vi "_시리얼 데이타 전송.vi"(2 "전송 문자열":string="FPGARX 0 1", 3 "시리얼 포트":refnum<visa-resource-name>) -> (0 "Processing Time(ms)":u32, 1 "송신 실패(T)":bool)   [LabVIEW 2015]
panel:
  out "에러 출력":errorcluster
  out "수신 문자열 버퍼":string
  out "수신 타이머 값":u32
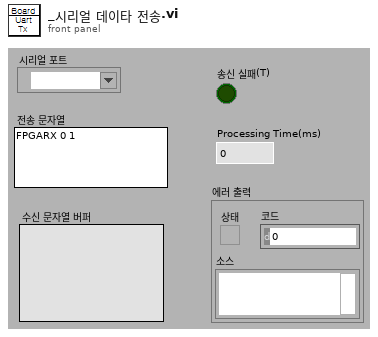
[diagram p1: front panel]
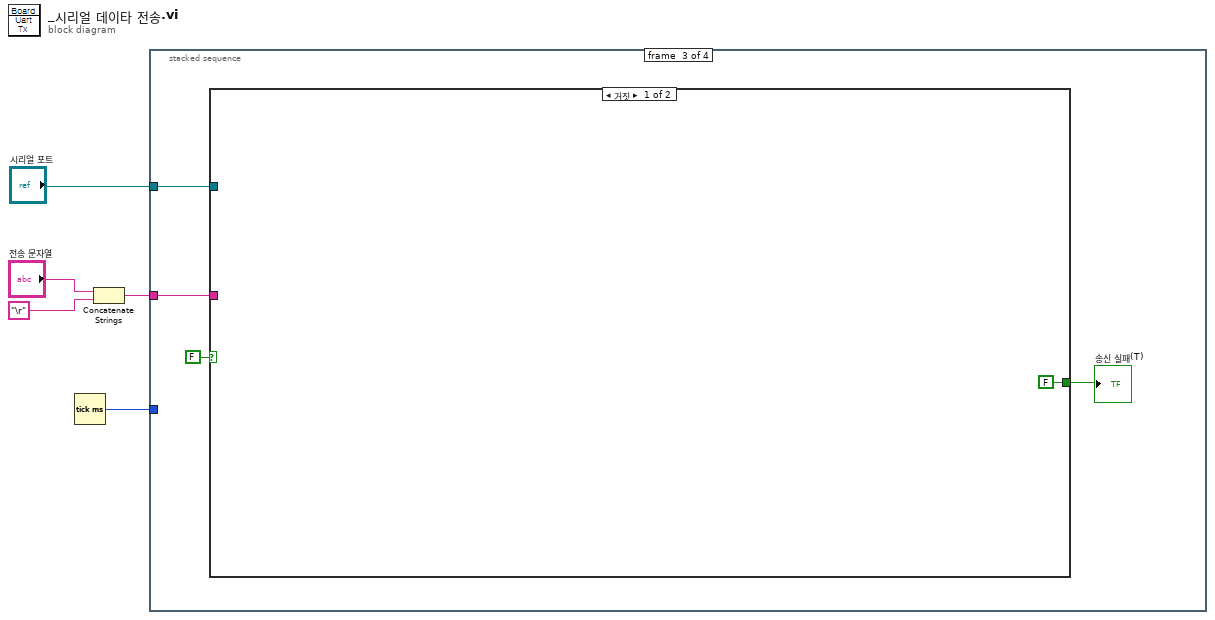
[diagram p0: block diagram]
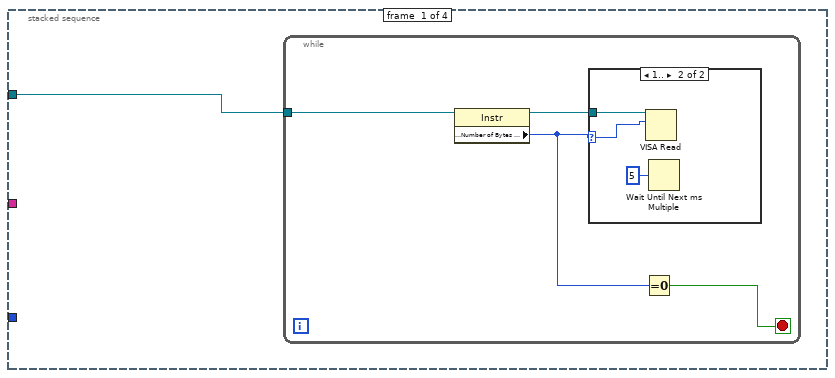
[diagram p2: hidden frame]
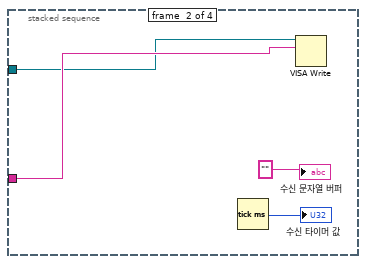
[diagram p4: hidden frame]
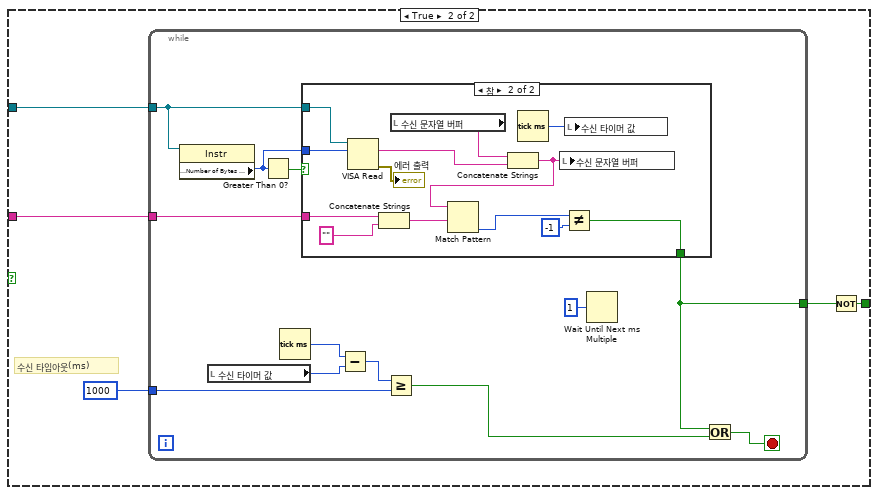
[diagram p5: hidden frame]
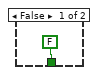
[diagram p6: hidden frame]
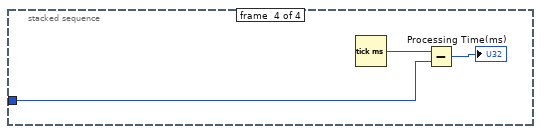
[diagram p7: hidden frame]
diagram:
  n1 = Tick Count (ms)() -> (millisecond timer value=w1:u32)
  n2 = Concatenate Strings("전송 문자열", "\r") -> (w3:string)
  n3 = stacked-sequence {
    tunnel: "시리얼 포트" -> [w6 w14 w21 _]
    tunnel: w3 -> [_ w17 w20 _]
    tunnel: w1 -> [_ _ _ w54]
    frame #0 {
      n4 = while {
        tunnel: w6 -> [w9]
        stop <- w8 stop-if-true
        n5 = property class="Instr"(reference=w9) -> (reference out=w10:refnum<visa-resource-name>, "Serial Settings:Number of Bytes at Serial Port"=w7:u32)  [unwired: 1 in, 1 out]
        n6 = case shown="1.." w7 {
          selector: w7 -> [_ w12]
          tunnel: w10 -> [_ w13]
          frame 0, Default {
          }
          frame 1.. {
            n7 = VISA Read(VISA resource name=w13, byte count=w12) -> ()  [unwired: 1 in, 4 out]
            n8 = Wait Until Next ms Multiple(millisecond multiple=u32 5 ("ms 배수")) -> ()  [unwired: 1 out]
          }
        }
        n9 = Equal To 0?(x=w7) -> (x = 0?=w8:bool)
      }
    }
    frame #1 {
      n10 = Tick Count (ms)() -> (millisecond timer value=→"수신 타이머 값":u32)
      n11 = VISA Write(VISA resource name=w14, write buffer=w17) -> ()  [unwired: 1 in, 3 out]
      "수신 문자열 버퍼" <- "" ("수신 문자열 버퍼")
    }
    frame #2 {
      n12 = case shown="거짓" FALSE {
        tunnel: w21 -> [_ w27]
        tunnel: w20 -> [_ w26]
        tunnel: [FALSE w23] -> w19
        frame False {
        }
        frame True {
          # "수신 타임아웃(ms)"
          n13 = while {
            tunnel: w27 -> [w39]
            tunnel: 1000 -> [w35]
            tunnel: w26 -> [w31]
            tunnel: [w29] -> w24
            stop <- w34 stop-if-true
            n14 = property class="Instr"(reference=w39) -> ("Serial Settings:Number of Bytes at Serial Port"=w32:u32)  [unwired: 1 in, 2 out]
            n15 = local read "수신 타이머 값"() -> (w36:u32)
            n16 = Greater Than 0?(x=w32) -> (x > 0?=w38:bool)
            n17 = Tick Count (ms)() -> (millisecond timer value=w37:u32)
            n18 = case shown="참" w38 {
              tunnel: w39 -> [_ w52]
              tunnel: [FALSE w46] -> w29
              tunnel: w32 -> [_ w45]
              tunnel: w31 -> [_ w43]
              frame False {
              }
              frame True {
                n19 = VISA Read(VISA resource name=w52, byte count=w45) -> (read buffer=w50:string, error out=→"에러 출력":errorcluster)  [unwired: 1 in, 2 out]
                n20 = Concatenate Strings(w43, "") -> (w42:string)
                n21 = local read "수신 문자열 버퍼"() -> (w53:string)
                n22 = Concatenate Strings(w53, w50) -> (w48:string)
                n23 = Match Pattern(string=w48, regular expression=w42) -> (offset past match=w47:i32)  [unwired: 1 in, 3 out]
                n24 = Tick Count (ms)() -> (millisecond timer value=w51:u32)
                n25 = local write "수신 문자열 버퍼"(w48) -> ()
                n26 = Not Equal?(x=w47, y=-1) -> (x != y?=w46:bool)
                n27 = local write "수신 타이머 값"(w51) -> ()
              }
            }
            n28 = Subtract(x=w37, y=w36) -> (x-y=w28:u32)
            n29 = Greater Or Equal?(x=w28, y=w35) -> (x >= y?=w33:bool)
            n30 = Wait Until Next ms Multiple(millisecond multiple=u32 1 ("ms 배수")) -> ()  [unwired: 1 out]
            n31 = Or(x=w29, y=w33) -> (x .or. y?=w34:bool)
          }
          n32 = Not(x=w24) -> (.not. x?=w23:bool)
        }
      }
      "송신 실패(T)" <- w19
    }
    frame #3 {
      n33 = Tick Count (ms)() -> (millisecond timer value=w56:u32)
      n34 = Subtract(x=w56, y=w54) -> (x-y=→"Processing Time(ms)":u32)
    }
  }
